vi "登陆界面.vi"() -> ()   [LabVIEW 2014]
uses:
  <vilib>/Utility/file.llb/Read From Spreadsheet File (string).vi
panel:
  out "学号与姓名表路径":path
  out "tips":string
  in  "用户名":string
  in  "密  码":string
  in  "退出":bool
  in  "登陆":bool
  in  "实验题目":u16(ring) items=["请下拉选择实验...", "X射线特征谱测量及Ｘ射线吸收", "α粒子能量损失", "β射线吸收", "γ能量测量实验", "放射性半衰期"]
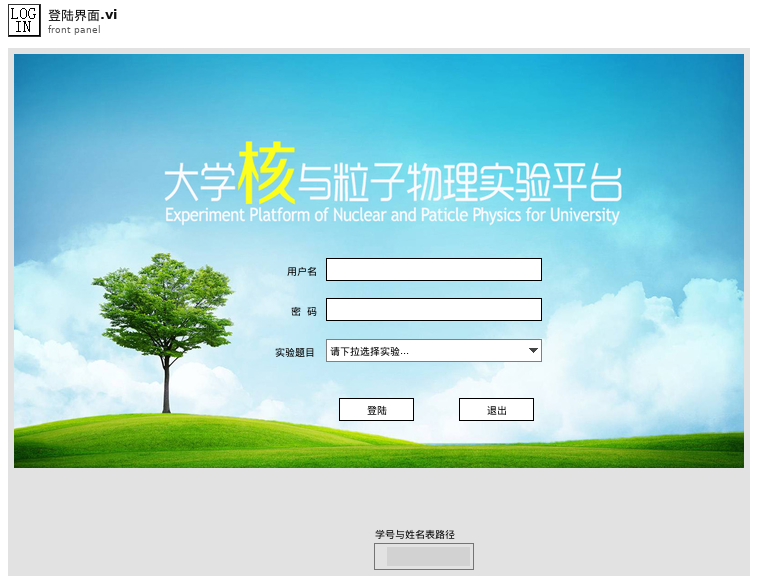
[diagram p1: front panel]
types:
  T1 = typedef "枚举常量_登陆界面.ctl" = enum16{"初始化", "等待用户输入", "信息匹配", "退出"}
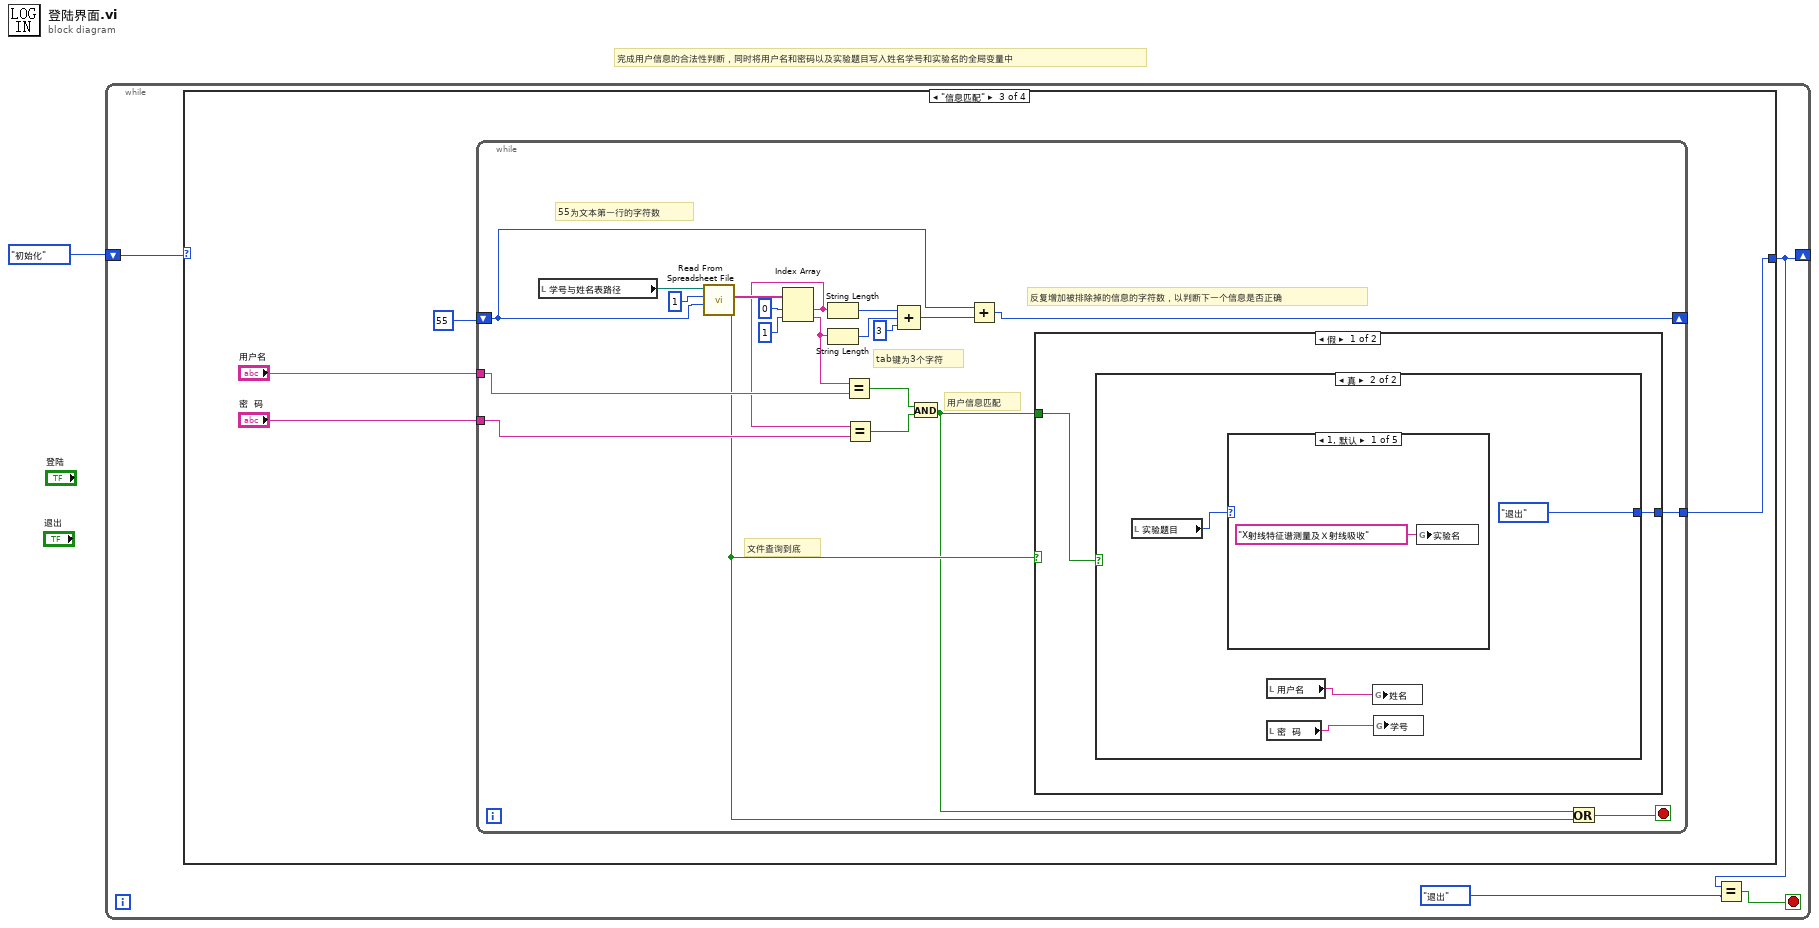
[diagram p0: block diagram]
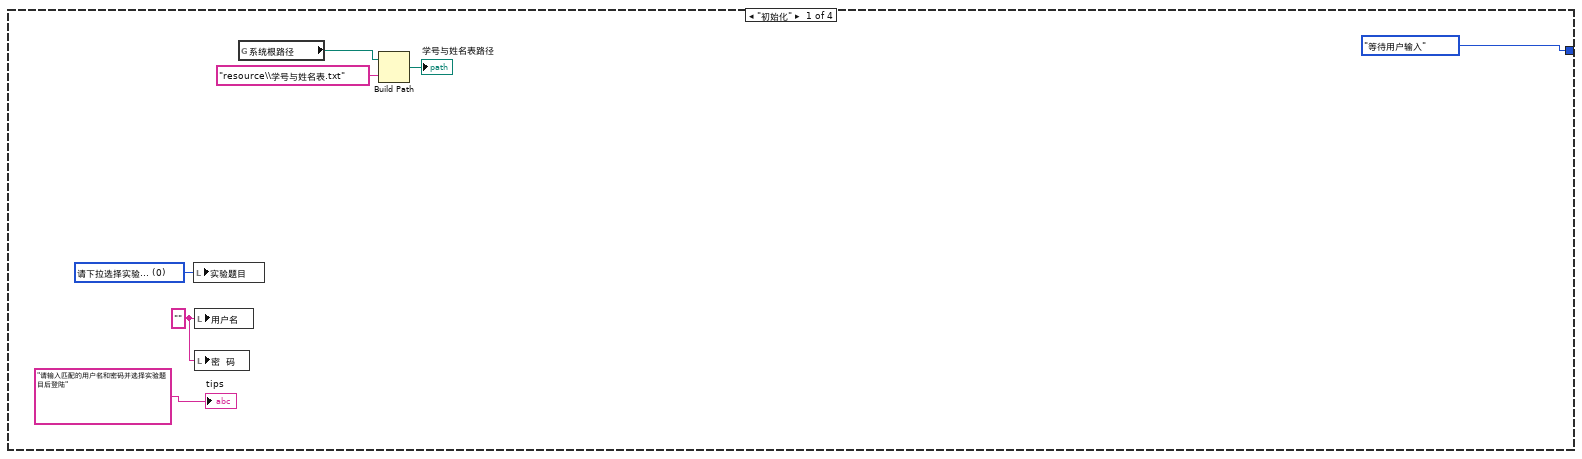
[diagram p2: hidden frame]
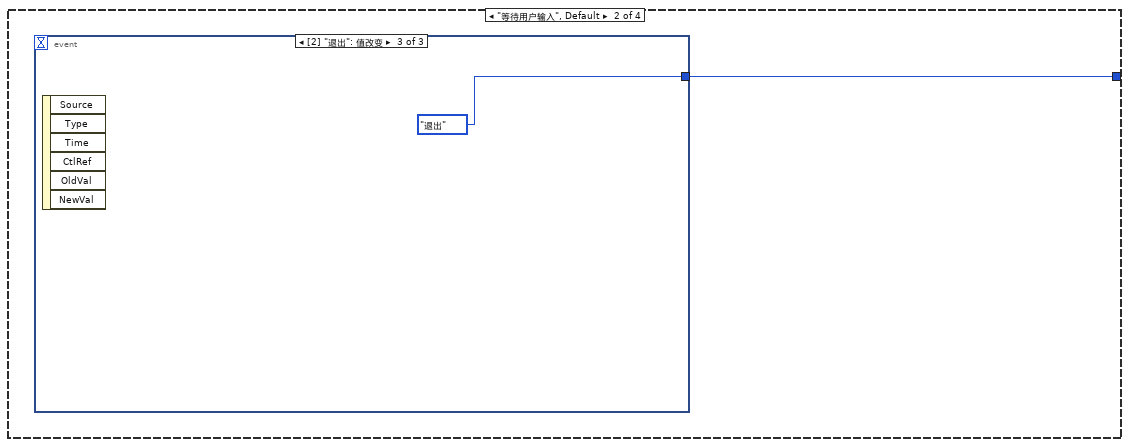
[diagram p3: hidden frame]
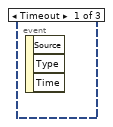
[diagram p4: hidden frame]
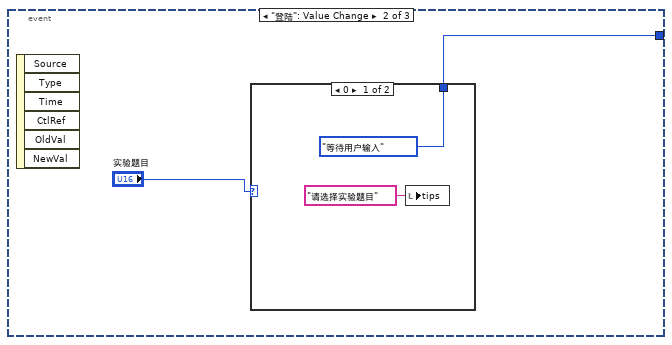
[diagram p5: hidden frame]
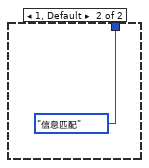
[diagram p6: hidden frame]
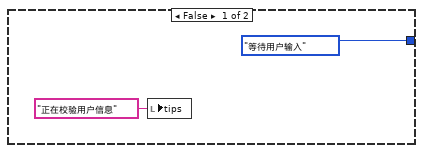
[diagram p7: hidden frame]
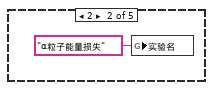
[diagram p8: hidden frame]
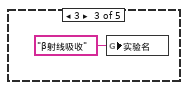
[diagram p9: hidden frame]
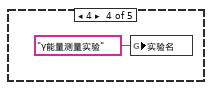
[diagram p10: hidden frame]
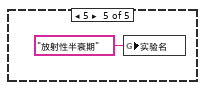
[diagram p11: hidden frame]
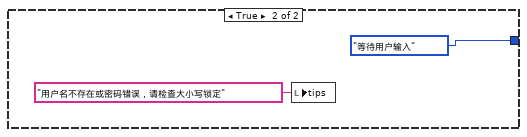
[diagram p12: hidden frame]
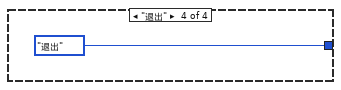
[diagram p13: hidden frame]
diagram:
  # "完成用户信息的合法性判断，同时将用户名和密码以及实验题目写入姓名学号和实验名的全局变量中"
  n1 = while {
    shift-right: [w2] -> _
    shift-left: 枚举常量_登陆界面."初始化" -> [w3]
    stop <- w4 stop-if-true
    n2 = case shown="\"信息匹配\"" w3 {
      tunnel: [枚举常量_登陆界面."等待用户输入" ("枚举") w13 w20 枚举常量_登陆界面."退出" ("枚举")] -> w2
      frame "初始化" {
        w11 = "" ("用户名")
        w12 = u16 0 items=["请下拉选择实验...", "X射线特征谱测量及Ｘ射线吸收", "α粒子能量损失", "β射线吸收", "γ能量测量实验", "放射性半衰期"] ("实验题目")
        n3 = local write "实验题目"(w12) -> ()
        n4 = local write "用户名"(w11) -> ()
        n5 = local write "密  码"(w11) -> ()
        n6 = global read "系统全局变量.vi" "系统根路径"() -> (w9:path)
        n7 = Build Path(base path=w9, name or relative path="resource\\学号与姓名表.txt" ("名称或相对路径")) -> (appended path=→"学号与姓名表路径":path)
        "tips" <- "请输入匹配的用户名和密码并选择实验题目后登陆"
      }
      frame "等待用户输入", Default {
        n8 = event shown="[2] \"退出\": 值改变" {
          selector: _ -> [_ _ _]
          dyn-events: _ -> [_ _ _]
          timeout: _ -> [_ _ _]
          tunnel: [_ w14 枚举常量_登陆界面."退出" ("枚举")] -> w13
          event Timeout {
            n9 = event-data() -> ()  [unwired: 1 in, 3 out]
          }
          event "登陆": Value Change {
            n10 = event-data() -> ()  [unwired: 1 in, 6 out]
            n11 = case shown="0" "实验题目" {
              tunnel: [枚举常量_登陆界面."等待用户输入" ("枚举") 枚举常量_登陆界面."信息匹配" ("枚举")] -> w14
              frame 0 {
                n12 = local write "tips"("请选择实验题目" ("tips")) -> ()
              }
              frame 1, Default {
              }
            }
          }
          event "退出": Value Change {
            n13 = event-data() -> ()  [unwired: 1 in, 6 out]
          }
        }
      }
      frame "信息匹配" {
        n14 = while {
          shift-right: [w34] -> _
          shift-left: 55 -> [w36]
          tunnel: "用户名" -> [w32]
          tunnel: "密  码" -> [w30]
          tunnel: [w24] -> w20
          stop <- w27 stop-if-true
          # "用户信息匹配"
          # "文件查询到底"
          # "反复增加被排除掉的信息的字符数，以判断下一个信息是否正确"
          # "55为文本第一行的字符数"
          # "tab键为3个字符"
          n15 = local read "学号与姓名表路径"() -> (w37:path)
          n16 = call-poly <vilib>:"Read From Spreadsheet File.vi"("start of read offset (chars.:0)"=w36, "number of rows (all:-1)"=1, "file path (dialog if empty)"=w37) -> ("EOF?"=w26:bool, "first row"=w43:string[])  [unwired: 4 in, 3 out]
          n17 = Index Array(array=w43, index #1=0 ("索引"), index #2=1 ("索引")) -> (element #1=w31:string, element #2=w33:string)
          n18 = String Length(string=w31) -> (length=w40:i32)
          n19 = String Length(string=w33) -> (length=w39:i32)
          n20 = Equal?(x=w33, y=w32) -> (x = y?=w29:bool)
          n21 = Equal?(x=w31, y=w30) -> (x = y?=w28:bool)
          n22 = Compound Arithmetic op=ADD(w40, w39, 3 ("值")) -> (w35:i32)
          n23 = And(x=w29, y=w28) -> (x .and. y?=w25:bool)
          n24 = Add(x=w36, y=w35) -> (x+y=w34:i32)
          n25 = case shown="假" w26 {
            tunnel: w25 -> [w46 _]
            tunnel: [w45 枚举常量_登陆界面."等待用户输入" ("枚举")] -> w24
            frame False {
              n26 = case shown="真" w46 {
                tunnel: [枚举常量_登陆界面."等待用户输入" ("枚举") 枚举常量_登陆界面."退出" ("枚举")] -> w45
                frame False {
                  n27 = local write "tips"("正在校验用户信息" ("tips")) -> ()
                }
                frame True {
                  n28 = local read "实验题目"() -> (w49:u16)
                  n29 = case shown="1, 默认" w49 {
                    frame 1, Default {
                      n30 = global write "系统全局变量.vi" "实验名"("X射线特征谱测量及Ｘ射线吸收" ("实验名")) -> ()
                    }
                    frame 2 {
                      n31 = global write "系统全局变量.vi" "实验名"("α粒子能量损失" ("实验名")) -> ()
                    }
                    frame 3 {
                      n32 = global write "系统全局变量.vi" "实验名"("β射线吸收" ("实验名")) -> ()
                    }
                    frame 4 {
                      n33 = global write "系统全局变量.vi" "实验名"("γ能量测量实验" ("实验名")) -> ()
                    }
                    frame 5 {
                      n34 = global write "系统全局变量.vi" "实验名"("放射性半衰期" ("实验名")) -> ()
                    }
                  }
                  n35 = local read "用户名"() -> (w51:string)
                  n36 = local read "密  码"() -> (w50:string)
                  n37 = global write "系统全局变量.vi" "姓名"(w51) -> ()
                  n38 = global write "系统全局变量.vi" "学号"(w50) -> ()
                }
              }
            }
            frame True {
              n39 = local write "tips"("用户名不存在或密码错误，请检查大小写锁定" ("tips")) -> ()
            }
          }
          n40 = Or(x=w25, y=w26) -> (x .or. y?=w27:bool)
        }
      }
      frame "退出" {
      }
    }
    n41 = Equal?(x=w2, y=枚举常量_登陆界面."退出" ("枚举")) -> (x = y?=w4:bool)
  }
